vi "VerifConfigState.vi"(8 "error in (no error)":errorcluster, 11 "Instrument in":refnum<class "Instrument.lvclass">) -> (0 "error out":errorcluster, 3 "Instrument out":refnum<class "Instrument.lvclass">)   [LabVIEW 2018, in "Instrument.lvclass"]
uses:
  Instrument.lvclass
  Instrument.lvclass/Instrument.ctl
  Device/Optics/Opt_Continuous/Opt_Continuous.lvclass
  Device/Optics/Opt_Selector/Opt_Selector.lvclass
  StateMachine/State Machine.lvclass
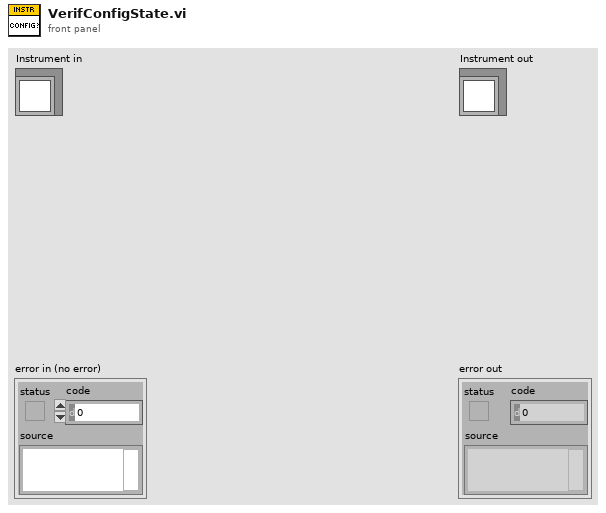
[diagram p1: front panel]
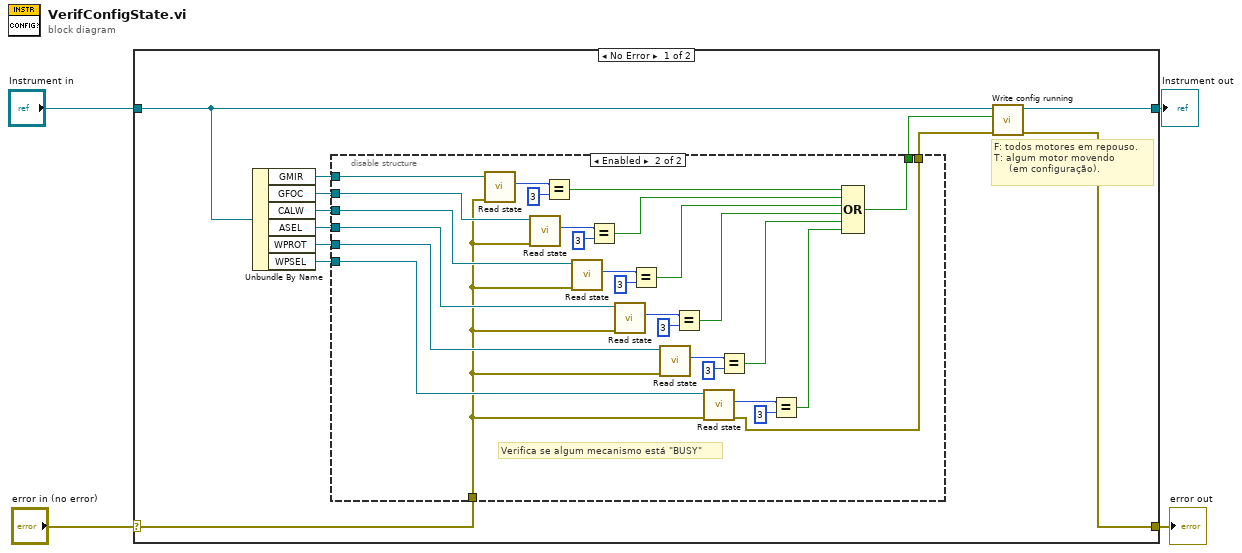
[diagram p0: block diagram]
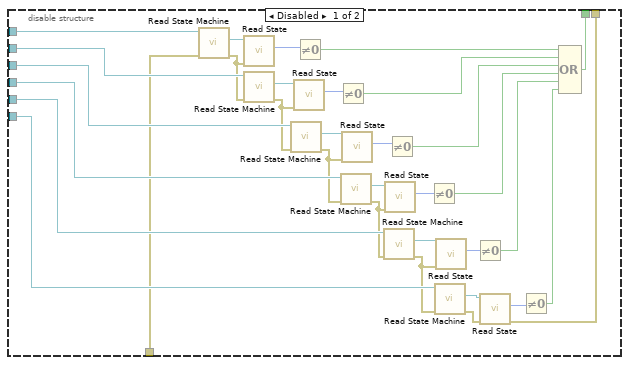
[diagram p2: hidden frame]
diagram:
  n1 = case shown="No Error" "error in (no error)" {
    selector: "error in (no error)" -> [w7 w78]
    tunnel: [w5 w78] -> w3
    tunnel: [w8 w77] -> w1
    tunnel: "Instrument in" -> [w10 w77]
    frame No Error {
      # "F: todos motores em repouso.\nT: algum motor movendo \n     (em configuração)."
      n2 = Unbundle By Name(w10) -> ("GMIR"=w16:refnum<class "Opt_Continuous.lvclass">, "GFOC"=w15:refnum<class "Opt_Continuous.lvclass">, "CALW"=w14:refnum<class "Opt_Selector.lvclass">, "ASEL"=w13:refnum<class "Opt_Selector.lvclass">, "WPROT"=w12:refnum<class "Opt_Selector.lvclass">, "WPSEL"=w11:refnum<class "Opt_Selector.lvclass">)
      n3 = disable-structure shown="Enabled" {
        disable-tunnel: w16 -> [w49 w74]
        disable-tunnel: w15 -> [w48 w63]
        disable-tunnel: w14 -> [w47 w62]
        disable-tunnel: w13 -> [w46 w61]
        disable-tunnel: w12 -> [w45 w60]
        disable-tunnel: w11 -> [w44 w59]
        disable-tunnel: [w25 w52] -> w9
        disable-tunnel: w7 -> [w24 w51]
        disable-tunnel: [w17 w50] -> w6
        frame Disabled {
          n4 = call-dynamic "Read State Machine.vi"("error in (no error)"=w24, "Device in"=w49) -> ("error out"=w23:errorcluster, "State Machine.lvclass"=w43:refnum<class "State Machine.lvclass">)  [unwired: 7 in, 1 out]
          n5 = call-dynamic "Read State.vi"("error in (no error)"=w23, "State Machine in"=w43) -> ("State"=w37:i32)  [unwired: 7 in, 2 out]
          n6 = call-dynamic "Read State Machine.vi"("error in (no error)"=w23, "Device in"=w48) -> ("error out"=w22:errorcluster, "State Machine.lvclass"=w42:refnum<class "State Machine.lvclass">)  [unwired: 7 in, 1 out]
          n7 = call-dynamic "Read State Machine.vi"("error in (no error)"=w22, "Device in"=w47) -> ("error out"=w21:errorcluster, "State Machine.lvclass"=w41:refnum<class "State Machine.lvclass">)  [unwired: 7 in, 1 out]
          n8 = call-dynamic "Read State.vi"("error in (no error)"=w22, "State Machine in"=w42) -> ("State"=w36:i32)  [unwired: 7 in, 2 out]
          n9 = Not Equal To 0?(x=w37) -> (x != 0?=w31:bool)
          n10 = Not Equal To 0?(x=w36) -> (x != 0?=w30:bool)
          n11 = call-dynamic "Read State Machine.vi"("error in (no error)"=w21, "Device in"=w46) -> ("error out"=w20:errorcluster, "State Machine.lvclass"=w40:refnum<class "State Machine.lvclass">)  [unwired: 7 in, 1 out]
          n12 = call-dynamic "Read State.vi"("error in (no error)"=w21, "State Machine in"=w41) -> ("State"=w35:i32)  [unwired: 7 in, 2 out]
          n13 = call-dynamic "Read State Machine.vi"("error in (no error)"=w20, "Device in"=w45) -> ("error out"=w19:errorcluster, "State Machine.lvclass"=w39:refnum<class "State Machine.lvclass">)  [unwired: 7 in, 1 out]
          n14 = call-dynamic "Read State.vi"("error in (no error)"=w20, "State Machine in"=w40) -> ("State"=w34:i32)  [unwired: 7 in, 2 out]
          n15 = Not Equal To 0?(x=w35) -> (x != 0?=w29:bool)
          n16 = Not Equal To 0?(x=w34) -> (x != 0?=w28:bool)
          n17 = call-dynamic "Read State Machine.vi"("error in (no error)"=w19, "Device in"=w44) -> ("error out"=w18:errorcluster, "State Machine.lvclass"=w38:refnum<class "State Machine.lvclass">)  [unwired: 7 in, 1 out]
          n18 = call-dynamic "Read State.vi"("error in (no error)"=w19, "State Machine in"=w39) -> ("State"=w33:i32)  [unwired: 7 in, 2 out]
          n19 = Not Equal To 0?(x=w33) -> (x != 0?=w27:bool)
          n20 = call-dynamic "Read State.vi"("error in (no error)"=w18, "State Machine in"=w38) -> ("error out"=w17:errorcluster, "State"=w32:i32)  [unwired: 7 in, 1 out]
          n21 = Not Equal To 0?(x=w32) -> (x != 0?=w26:bool)
          n22 = Compound Arithmetic op=OR(w31, w30, w29, w28, w27, w26) -> (w25:bool)
        }
        frame Enabled {
          # "Verifica se algum mecanismo está \"BUSY\""
          n23 = call-dynamic "Read state.vi"("error in (no error)"=w51, "Optics in"=w74) -> ("state"=w76:u8)  [unwired: 7 in, 2 out]
          n24 = call-dynamic "Read state.vi"("error in (no error)"=w51, "Optics in"=w63) -> ("state"=w73:u8)  [unwired: 7 in, 2 out]
          n25 = Equal?(x=w76, y=u8 3) -> (x = y?=w58:bool)
          n26 = call-dynamic "Read state.vi"("error in (no error)"=w51, "Optics in"=w62) -> ("state"=w71:u8)  [unwired: 7 in, 2 out]
          n27 = Equal?(x=w73, y=u8 3) -> (x = y?=w57:bool)
          n28 = call-dynamic "Read state.vi"("error in (no error)"=w51, "Optics in"=w61) -> ("state"=w69:u8)  [unwired: 7 in, 2 out]
          n29 = Equal?(x=w71, y=u8 3) -> (x = y?=w56:bool)
          n30 = call-dynamic "Read state.vi"("error in (no error)"=w51, "Optics in"=w60) -> ("state"=w67:u8)  [unwired: 7 in, 2 out]
          n31 = Equal?(x=w69, y=u8 3) -> (x = y?=w55:bool)
          n32 = call-dynamic "Read state.vi"("error in (no error)"=w51, "Optics in"=w59) -> ("error out"=w50:errorcluster, "state"=w65:u8)  [unwired: 7 in, 1 out]
          n33 = Equal?(x=w67, y=u8 3) -> (x = y?=w54:bool)
          n34 = Equal?(x=w65, y=u8 3) -> (x = y?=w53:bool)
          n35 = Compound Arithmetic op=OR(w58, w57, w56, w55, w54, w53) -> (w52:bool)
        }
      }
      n36 = call-dynamic "Write config running.vi"("error in (no error)"=w6, "config running"=w9, "Server in"=w10) -> ("error out"=w5:errorcluster, "Server out"=w8:refnum<class "Instrument.lvclass">)  [unwired: 7 in]
    }
    frame Error {
    }
  }
  "error out" <- w3
  "Instrument out" <- w1
